vi "InitializeLaser.vi"(8 "error in":errorcluster, 10 "ON/OFF":bool, 11 "VISA resource name in":refnum<visa-resource-name>) -> (0 "error out":errorcluster, 1 "Fmin":dbl, 2 "Fmax":dbl, 3 "VISA resource name out":refnum<visa-resource-name>, 4 "Tmax":dbl, 5 "SN:":string, 6 "Tmin":dbl, 7 "Лазер: ID:":string)   [LabVIEW 2014]
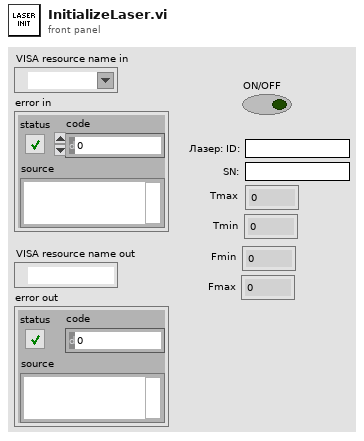
[diagram p1: front panel]
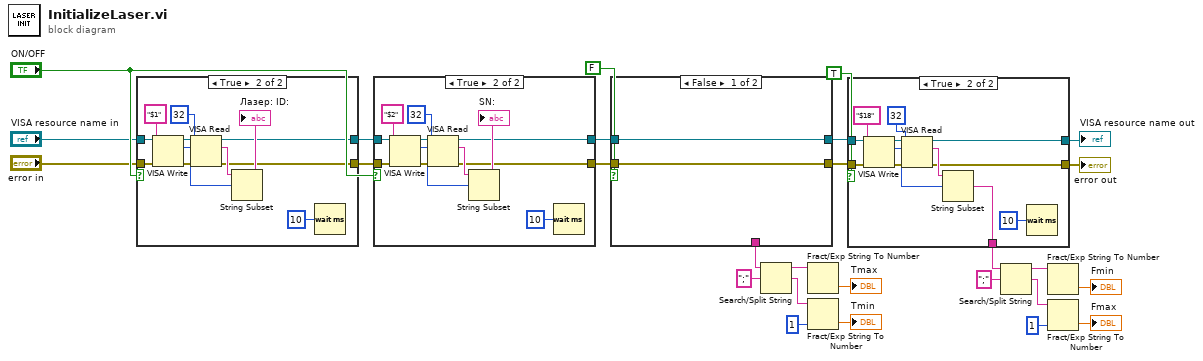
[diagram p0: block diagram]
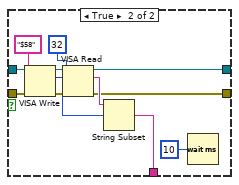
[diagram p3: hidden frame]
diagram:
  n1 = case shown="True" "ON/OFF" {
    tunnel: "VISA resource name in" -> [w29 w39]
    tunnel: "error in" -> [w28 w38]
    tunnel: [w29 w31] -> w23
    tunnel: [w28 w30] -> w22
    frame False {
    }
    frame True {
      n2 = VISA Write(VISA resource name=w39, write buffer="$1", error in (no error)=w38) -> (VISA resource name out=w40:refnum<visa-resource-name>, return count=w34:u32, error out=w41:errorcluster)
      n3 = VISA Read(VISA resource name=w40, byte count=u32 32, error in (no error)=w41) -> (VISA resource name out=w31:refnum<visa-resource-name>, read buffer=w32:string, error out=w30:errorcluster)  [unwired: 1 out]
      n4 = String Subset(string=w32, offset (0)=w34) -> (substring=→"Лазер: ID:":string)  [unwired: 1 in]
      n5 = Wait (ms)(milliseconds to wait=u32 10) -> ()  [unwired: 1 out]
    }
  }
  n6 = case shown="True" "ON/OFF" {
    tunnel: w23 -> [w43 w53]
    tunnel: w22 -> [w42 w52]
    tunnel: [w43 w45] -> w21
    tunnel: [w42 w44] -> w20
    frame False {
    }
    frame True {
      n7 = VISA Write(VISA resource name=w53, write buffer="$2", error in (no error)=w52) -> (VISA resource name out=w54:refnum<visa-resource-name>, return count=w48:u32, error out=w55:errorcluster)
      n8 = VISA Read(VISA resource name=w54, byte count=u32 32, error in (no error)=w55) -> (VISA resource name out=w45:refnum<visa-resource-name>, read buffer=w47:string, error out=w44:errorcluster)  [unwired: 1 out]
      n9 = String Subset(string=w47, offset (0)=w48) -> (substring=→"SN:":string)  [unwired: 1 in]
      n10 = Wait (ms)(milliseconds to wait=u32 10) -> ()  [unwired: 1 out]
    }
  }
  n11 = case shown="False" FALSE {
    tunnel: w21 -> [w57 w67]
    tunnel: w20 -> [w56 w66]
    tunnel: [w57 w59] -> w4
    tunnel: [w56 w58] -> w3
    tunnel: [_ w62] -> w19
    frame False {
    }
    frame True {
      n12 = VISA Write(VISA resource name=w67, write buffer="$58", error in (no error)=w66) -> (VISA resource name out=w68:refnum<visa-resource-name>, return count=w61:u32, error out=w69:errorcluster)
      n13 = VISA Read(VISA resource name=w68, byte count=u32 32, error in (no error)=w69) -> (VISA resource name out=w59:refnum<visa-resource-name>, read buffer=w60:string, error out=w58:errorcluster)  [unwired: 1 out]
      n14 = String Subset(string=w60, offset (0)=w61) -> (substring=w62:string)  [unwired: 1 in]
      n15 = Wait (ms)(milliseconds to wait=u32 10) -> ()  [unwired: 1 out]
    }
  }
  n16 = Search/Split String(string=w19, search string/char (-)=";") -> (substring before match=w26:string, match + rest of string=w25:string)  [unwired: 1 in, 1 out]
  n17 = Fract/Exp String To Number(string=w26) -> (number=→"Tmax":dbl)  [unwired: 3 in, 1 out]
  n18 = Fract/Exp String To Number(string=w25, offset=1) -> (number=→"Tmin":dbl)  [unwired: 2 in, 1 out]
  n19 = case shown="True" TRUE {
    tunnel: w4 -> [w71 w81]
    tunnel: w3 -> [w70 w80]
    tunnel: [w71 w73] -> w2
    tunnel: [w70 w72] -> w1
    tunnel: [_ w76] -> w8
    frame False {
    }
    frame True {
      n20 = VISA Write(VISA resource name=w81, write buffer="$18", error in (no error)=w80) -> (VISA resource name out=w82:refnum<visa-resource-name>, return count=w75:u32, error out=w83:errorcluster)
      n21 = VISA Read(VISA resource name=w82, byte count=u32 32, error in (no error)=w83) -> (VISA resource name out=w73:refnum<visa-resource-name>, read buffer=w74:string, error out=w72:errorcluster)  [unwired: 1 out]
      n22 = String Subset(string=w74, offset (0)=w75) -> (substring=w76:string)  [unwired: 1 in]
      n23 = Wait (ms)(milliseconds to wait=u32 10) -> ()  [unwired: 1 out]
    }
  }
  "VISA resource name out" <- w2
  "error out" <- w1
  n24 = Search/Split String(string=w8, search string/char (-)=";") -> (substring before match=w11:string, match + rest of string=w10:string)  [unwired: 1 in, 1 out]
  n25 = Fract/Exp String To Number(string=w11) -> (number=→"Fmin":dbl)  [unwired: 3 in, 1 out]
  n26 = Fract/Exp String To Number(string=w10, offset=1) -> (number=→"Fmax":dbl)  [unwired: 2 in, 1 out]
